vi "Leaf_Init.vi"(8 "error in (no error)":errorcluster, 11 "Object in":refnum<class "Leaf.lvclass">) -> (0 "error out":errorcluster, 3 "object out":refnum<class "Leaf.lvclass">)   [LabVIEW 2019, in "Leaf.lvclass"]
uses:
  Leaf.lvclass
  C:/Program Files (x86)/National Instruments/LabVIEW 2019/examples/Open_GDS/GDS/InterfaceByViServer/Sub_class/Sub.lvclass
  Leaf.lvclass/Leaf.ctl
  Sub_class/Sub.lvclass
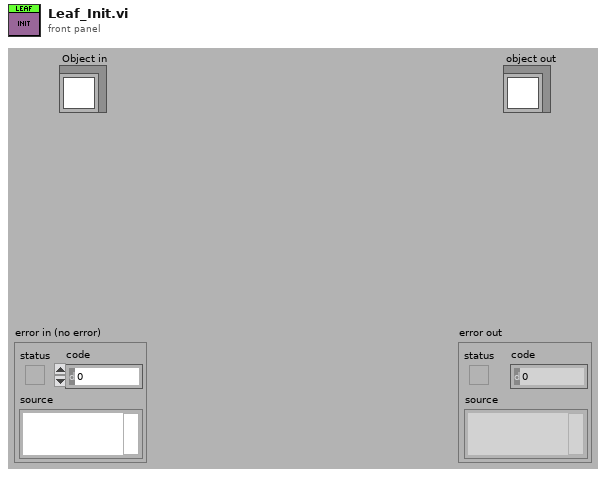
[diagram p1: front panel]
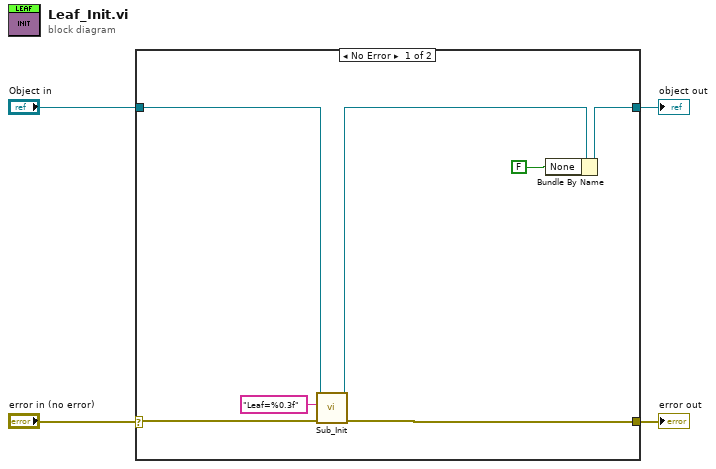
[diagram p0: block diagram]
diagram:
  n1 = case shown="No Error" "error in (no error)" {
    selector: "error in (no error)" -> [w9 w12]
    tunnel: [w11 w13] -> w4
    tunnel: "Object in" -> [w7 w13]
    tunnel: [w8 w12] -> w1
    frame No Error {
      n2 = call "Sub_Init.vi"("error in (no error)"=w9, "String"="Leaf=%0.3f", "Object in"=w7) -> ("error out"=w8:errorcluster, "object out"=w6:refnum<class "Leaf.lvclass">)  [unwired: 7 in]
      n3 = Bundle By Name(cluster=w6, "None"=FALSE) -> (w11:refnum<class "Leaf.lvclass">)
    }
    frame Error {
    }
  }
  "object out" <- w4
  "error out" <- w1
